vi "SaveData.vi"(7 "LabVIEW Web Service Request":refnum<class "Web Request.lvclass">, 10 "MeasurementValue":dbl, 11 "MeasurementName":string) -> ()   [LabVIEW 2015]
uses:
  <vilib>/wsapi/Web Request.lvclass
panel:
  out "Error out":errorcluster
  # "Use the Web Service Request input terminal to call the VIs on the Web Services palette. Do not remove it from the connector pane unless you don't need access to the palette."
  # "Each additional control wired to the connector pane will be available as an input in the URL. To include an indicator in terminal-mode output (the default setting), it must also be wired to the connector pane."
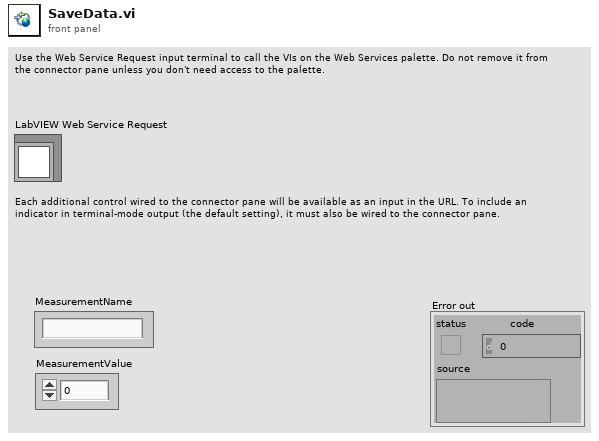
[diagram p1: front panel]
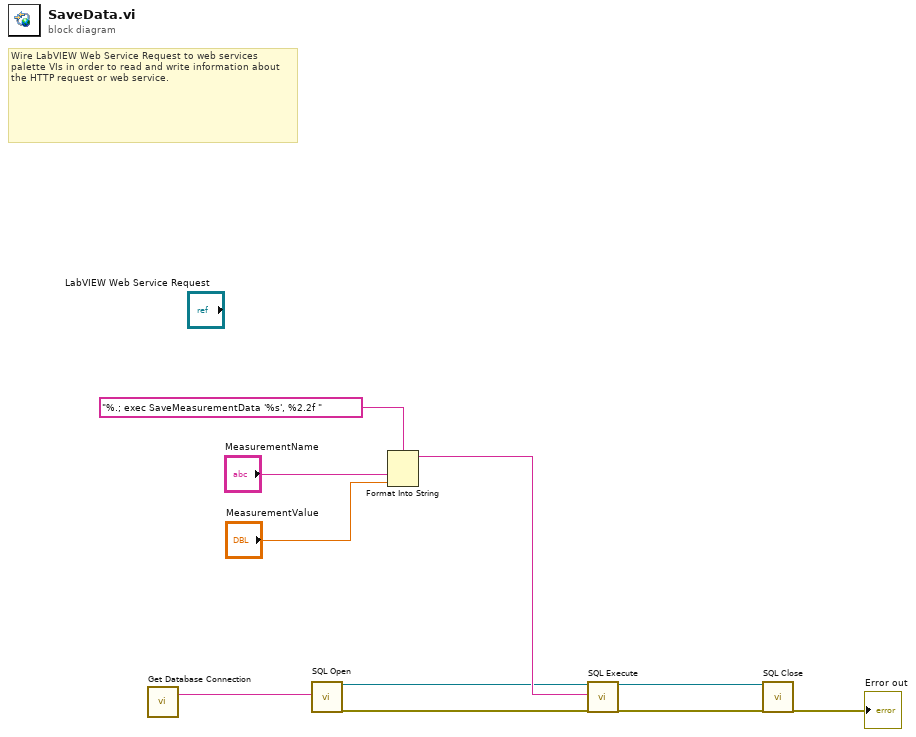
[diagram p0: block diagram]
diagram:
  # "Wire LabVIEW Web Service Request to web services palette VIs in order to read and write information about the HTTP request or web service."
  n1 = call "Get Database Connection.vi"() -> ("Database  Connection String"=w2:string)  [unwired: 2 in, 1 out]
  n2 = call <vilib>:"SQL Open.vi"("ConnectionString In"=w2) -> ("Connection Out"=w8:refnum<k7>, "Error out"=w4:errorcluster)  [unwired: 17 in]
  n3 = Format Into String "Format Into String"(format string="%.; exec SaveMeasurementData '%s', %2.2f ", "MeasurementName", "MeasurementValue") -> (resulting string=w9:string)  [unwired: 2 in, 1 out]
  n4 = call <vilib>:"SQL Execute.vi"("Connection In"=w8, "SQL Query"=w9, "Error in (no error)"=w4) -> ("Connection Out"=w5:refnum<k7>, "Error out"=w3:errorcluster)  [unwired: 15 in]
  n5 = call <vilib>:"SQL Close.vi"("Connection In"=w5, "Error in (no error)"=w3) -> ("Error out"=→"Error out":errorcluster)  [unwired: 17 in]
